vi "CheckShot2Invader.vi"(6 "IntensityArray_IN":u8[][](array[numeric]), 7 "InvaderPosArray_IN":T1, 11 "ShotArray_IN":T3[](array[typedef])) -> (3 "ShotArray_OUT":T3[](array[typedef]), 4 "IntensityArray_OUT":u8[][](array[numeric]), 5 "InvaderPosArray_OUT":T1)   [LabVIEW 2019]
uses:
  InvaderPositionArray.ctl
  move_dir_lr.ctl
  ShotCluster.ctl
  move_dir_ud.ctl
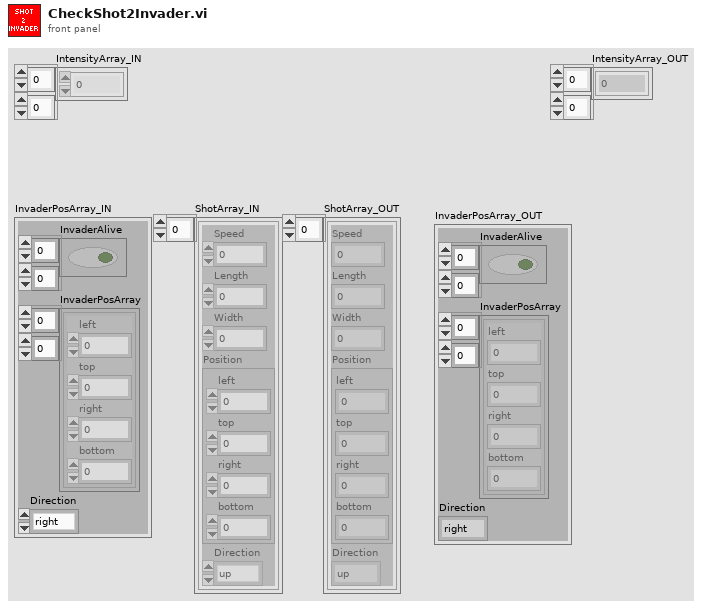
[diagram p1: front panel]
types:
  T1 = typedef "InvaderPositionArray.ctl" = cluster{"InvaderAlive":bool[][], "InvaderPosArray":cluster{"left":i16, "top":i16, "right":i16, "bottom":i16}[][], "Direction":T2}
  T2 = typedef "move_dir_lr.ctl" = enum16{"right", "left"}
  T3 = typedef "ShotCluster.ctl" = cluster{"Speed":u32, "Length":u32, "Width":u32, "Position":cluster{"left":i16, "top":i16, "right":i16, "bottom":i16}, "Direction":T4}
  T4 = typedef "move_dir_ud.ctl" = enum16{"up", "down"}
  T5 = cluster{"left":i16, "top":i16, "right":i16, "bottom":i16}[]
  T6 = cluster{"left":i16, "top":i16, "right":i16, "bottom":i16}
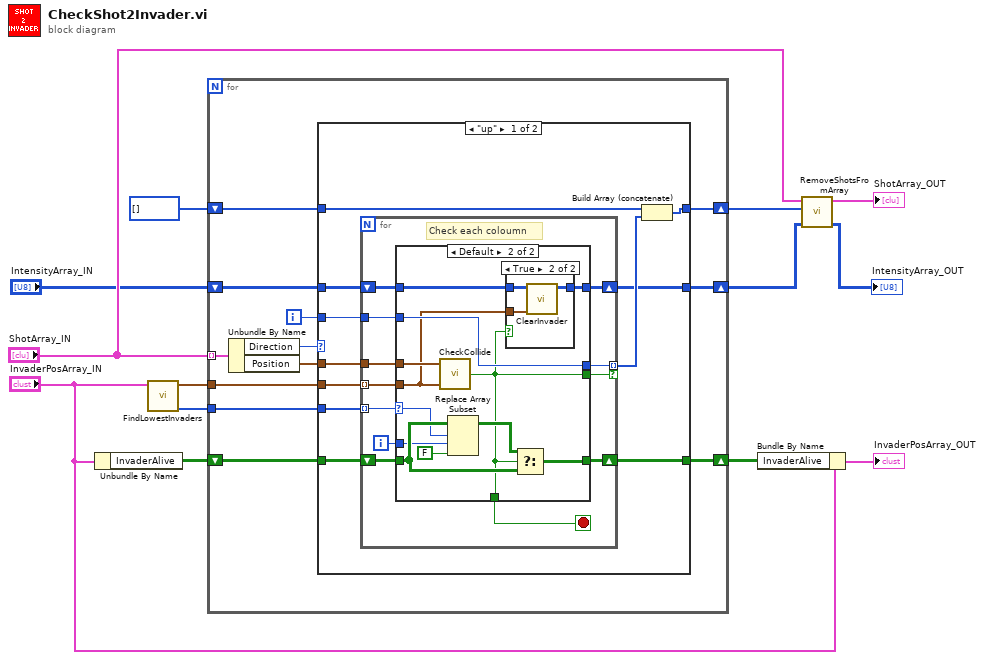
[diagram p0: block diagram]
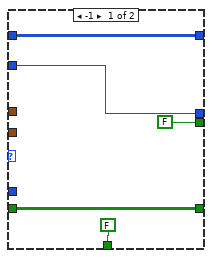
[diagram p2: hidden frame]
diagram:
  n1 = Unbundle By Name("InvaderPosArray_IN") -> ("InvaderAlive"=w12:bool[][])
  n2 = call "FindLowestInvaders.vi"("InvaderPosArray_IN"="InvaderPosArray_IN") -> ("LowestRowIndexes"=w4:i32[], "LowestPositions"=w13:T5)  [unwired: 9 in]
  n3 = for {
    tunnel: "ShotArray_IN" -> [w25] mode=indexing
    tunnel: w13 -> [w21]
    shift-right: [w20] -> w10
    shift-left: w12 -> [w23]
    shift-right: [w17] -> w3
    shift-left: i32[] [] -> [w18]
    shift-right: [w14] -> w2
    shift-left: "IntensityArray_IN" -> [w15]
    tunnel: w4 -> [w16]
    i -> [w19]
    n4 = Unbundle By Name(w25) -> ("Direction"=w24:T4, "Position"=w22:T6)
    n5 = case shown="\"up\"" w24 {
      tunnel: w23 -> [w34 w72]
      tunnel: w22 -> [w36 _]
      tunnel: w21 -> [w35 _]
      tunnel: [w33 w72] -> w20
      tunnel: w19 -> [w32 _]
      tunnel: w18 -> [w31 w71]
      tunnel: [w29 w71] -> w17
      tunnel: w16 -> [w28 _]
      tunnel: w15 -> [w27 w70]
      tunnel: [w26 w70] -> w14
      frame "up" {
        n6 = for {
          tunnel: w36 -> [w48]
          tunnel: w35 -> [w47] mode=indexing
          shift-right: [w43] -> w33
          shift-left: w34 -> [w45]
          tunnel: w32 -> [w42]
          tunnel: [w41] -> w30 mode=indexing if=w40
          tunnel: w28 -> [w39] mode=indexing
          shift-right: [w37] -> w26
          shift-left: w27 -> [w38]
          i -> [w44]
          stop <- w46 stop-if-true
          # "Check each coloumn"
          n7 = case shown="Default" w39 {
            selector: w39 -> [_ w60]
            tunnel: w48 -> [_ w65]
            tunnel: w47 -> [_ w54]
            tunnel: [FALSE ("Collide") w57] -> w46
            tunnel: w45 -> [w52 w64]
            tunnel: w44 -> [_ w59]
            tunnel: [w52 w61] -> w43
            tunnel: w42 -> [w51 w58]
            tunnel: [w51 w58] -> w41
            tunnel: [FALSE ("Collide") w57] -> w40
            tunnel: w38 -> [w49 w56]
            tunnel: [w49 w55] -> w37
            frame -1 {
            }
            frame Default {
              n8 = call "CheckCollide.vi"("Rectangle2"=w54, "Rectangle1"=w65) -> ("Collide"=w57:bool)  [unwired: 3 in]
              n9 = Replace Array Subset(array=w64, new element=FALSE, index (row)=w60, index (col)=w59) -> (w62:bool[][])
              n10 = case shown="True" w57 {
                tunnel: w56 -> [w66 w69]
                tunnel: [w66 w68] -> w55
                tunnel: w54 -> [_ w67]
                frame False {
                }
                frame True {
                  n11 = call "ClearInvader.vi"("InvaderPosition"=w67, "IntensityArray_IN"=w69) -> ("IntensityArray_OUT"=w68:u8[][])  [unwired: 9 in]
                }
              }
              n12 = Select(t=w62, s=w57, f=w64) -> (s? t:f=w61:bool[][])
            }
          }
        }
        n13 = Build Array (concatenate)(w31, w30) -> (w29:i32[])
      }
      frame "down" {
      }
    }
  }
  n14 = Bundle By Name(cluster="InvaderPosArray_IN", "InvaderAlive"=w10) -> (→"InvaderPosArray_OUT":T1)
  n15 = call "RemoveShotsFromArray.vi"("IntensityArray_IN"=w2, "Indexes"=w3, "ShotArray_IN"="ShotArray_IN") -> ("IntensityArray_OUT"=→"IntensityArray_OUT":u8[][], "ShotArray_OUT"=→"ShotArray_OUT":T3[])  [unwired: 7 in]
